vi "GUI.vi"() -> ()   [LabVIEW 2018]
uses:
  <vilib>/Utility/file.llb/Write Delimited Spreadsheet (DBL).vi
panel:
  in  "backlash steps":i32=1000
  out "error out":errorcluster
  in  "Save data?":bool
  in  "file path (dialog if empty)":path
  in  "transpose? (no:F)":bool
  out "Latest Linescan":dbl[](graph)
  out "Intensity Graph":dbl[][](graph)
  in  "Calibration factor":dbl
  in  "Y Range":dbl
  in  "X Range":dbl
  in  "error in":errorcluster
  in  "Scan Rate":dbl
  in  "Y points":dbl
  in  "X points":dbl
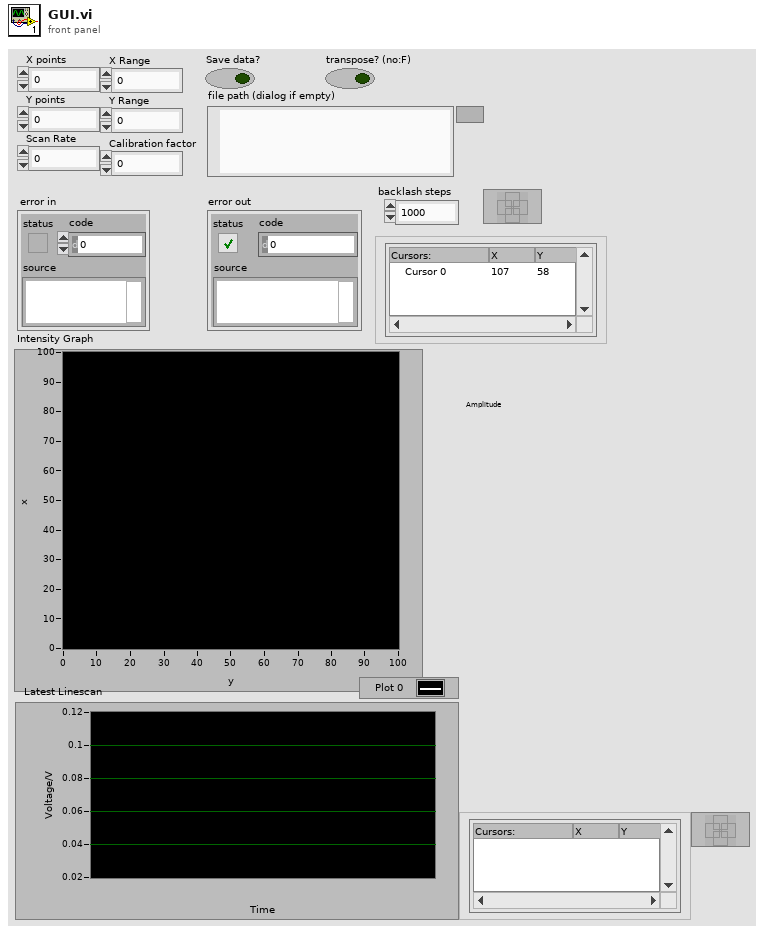
[diagram p1: front panel]
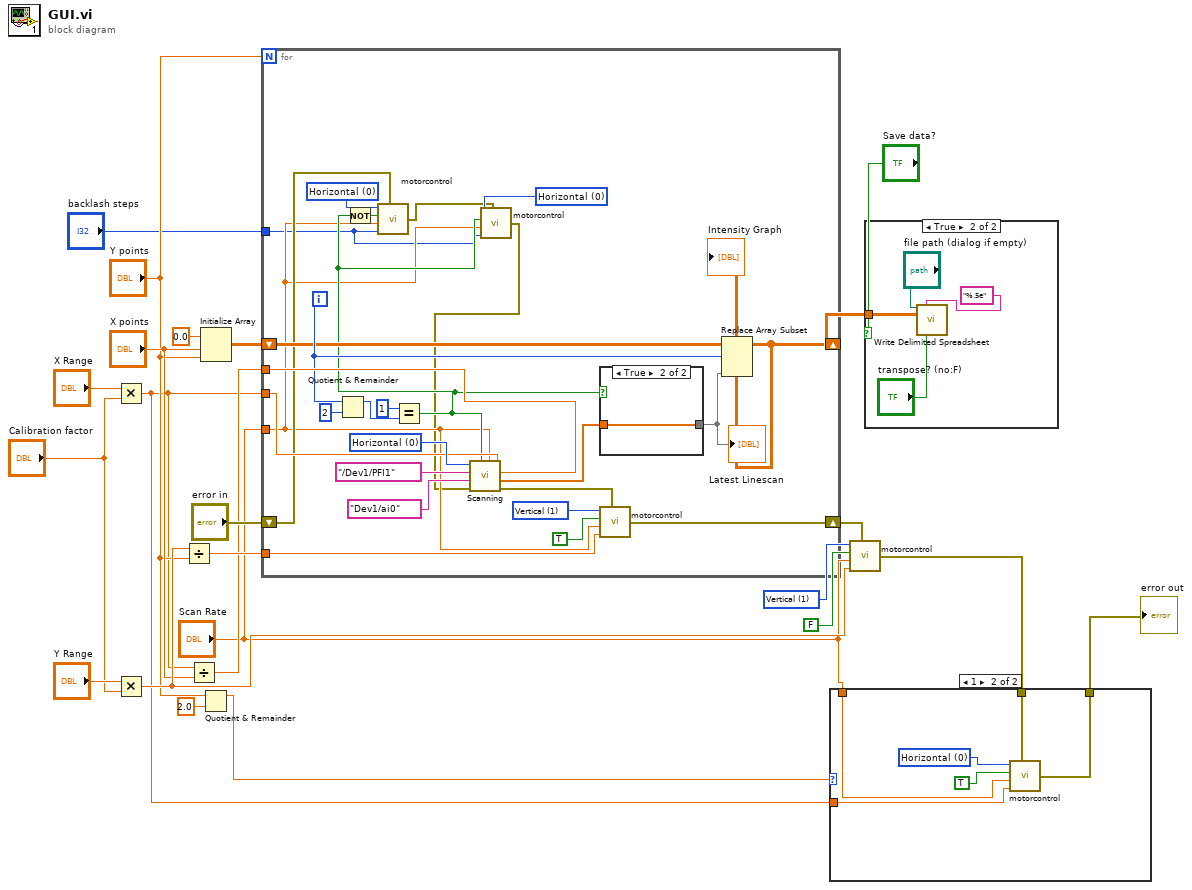
[diagram p0: block diagram]
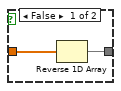
[diagram p4: hidden frame]
diagram:
  w20 = u16 1 items=["Horizontal", "Vertical"] ("Ring")
  n1 = Multiply(x="X Range", y="Calibration factor") -> (x*y=w4:dbl)
  n2 = Multiply(x="Y Range", y="Calibration factor") -> (x*y=w18:dbl)
  n3 = Divide(x=w18, y="Y points") -> (x/y=w15:dbl)
  n4 = Divide(x=w4, y="X points") -> (x/y=w14:dbl)
  n5 = Initialize Array(0.0 ("element"), "X points", "Y points") -> (w9:dbl[][])
  n6 = Quotient & Remainder(x="Y points", y=2.0) -> (x-y*floor(x/y)=w8:dbl)  [unwired: 1 out]
  n7 = for {
    N: "Y points" -> [_]
    tunnel: "Scan Rate" -> [w28]
    shift-right: [w42] -> w13
    shift-left: "error in" -> [w31]
    tunnel: w4 -> [w41]
    tunnel: w14 -> [w40]
    tunnel: w15 -> [w39]
    shift-right: [w37] -> w3
    shift-left: w9 -> [w36]
    tunnel: "backlash steps" -> [w24]
    i -> [w38]
    w27 = u16 0 items=["Horizontal", "Vertical"] ("Ring")
    w32 = u16 0 items=["Horizontal", "Vertical"] ("Ring")
    w45 = u16 1 items=["Horizontal", "Vertical"] ("Ring")
    w46 = u16 0 items=["Horizontal", "Vertical"] ("Motor")
    n8 = Quotient & Remainder(x=w38, y=2) -> (x-y*floor(x/y)=w35:i32)  [unwired: 1 out]
    n9 = Equal?(x=1, y=w35) -> (x = y?=w29:bool)
    n10 = Not(x=w29) -> (.not. x?=w30:bool)
    n11 = call "motorcontrol.vi"("Ring"=w32, "Direction"=w30, "Frequency"=w28, "# of steps"=w24, "error in"=w31) -> ("error out"=w25:errorcluster)
    n12 = call "motorcontrol.vi"("Ring"=w27, "Direction"=w29, "Frequency"=w28, "# of steps"=w24, "error in"=w25) -> ("error out"=w26:errorcluster)
    n13 = call "Scanning.vi"("Number of steps/point"=w40, "Number of steps/line"=w41, "Step rate"=w28, "Scan direction"=w29, "error in"=w26, "ADC signal channels"=tag "Dev1/ai0", "clock for ADC"=tag "/Dev1/PFI1", "Motor"=w46) -> ("error out"=w43:errorcluster, "Voltage Signal"=w34:dbl[])
    n14 = case shown="True" w29 {
      tunnel: w34 -> [w52 w53]
      tunnel: [w51 w53] -> w33
      frame False {
        n15 = Reverse 1D Array(array=w52) -> (reversed array=w51:dbl[])
      }
      frame True {
      }
    }
    "Latest Linescan" <- w33
    n16 = call "motorcontrol.vi"("Ring"=w45, "Direction"=TRUE, "Frequency"=w28, "# of steps"=w39, "error in"=w43) -> ("error out"=w42:errorcluster)
    n17 = Replace Array Subset(array=w36, new element=w33, index (row)=w38) -> (w37:dbl[][])  [unwired: 1 in]
    "Intensity Graph" <- w37
  }
  n18 = call "motorcontrol.vi"("Ring"=w20, "Direction"=FALSE, "Frequency"="Scan Rate", "# of steps"=w18, "error in"=w13) -> ("error out"=w7:errorcluster)
  n19 = case shown="1" w8 {
    tunnel: w7 -> [w54 w58]
    tunnel: [w54 w57] -> w6
    tunnel: "Scan Rate" -> [_ w56]
    tunnel: w4 -> [_ w55]
    frame 0, Default {
    }
    frame 1 {
      w60 = u16 0 items=["Horizontal", "Vertical"] ("Ring")
      n20 = call "motorcontrol.vi"("Ring"=w60, "Direction"=TRUE, "Frequency"=w56, "# of steps"=w55, "error in"=w58) -> ("error out"=w57:errorcluster)
    }
  }
  "error out" <- w6
  n21 = case shown="True" "Save data?" {
    tunnel: w3 -> [_ w61]
    frame False {
    }
    frame True {
      n22 = call-poly <vilib>:"Write Delimited Spreadsheet.vi"("file path (dialog if empty)"="file path (dialog if empty)", "format (%.3f)"="%.5e", "2D data"=w61, "transpose? (no:F)"="transpose? (no:F)") -> ()  [unwired: 10 in, 2 out]
    }
  }
